vi "MoveXYAbs2.vi"(8 "error in (no error)":errorcluster, 9 "Y":dbl, 10 "X":dbl, 11 "connection ID":refnum<k5>) -> (0 "error out":errorcluster, 3 "connection ID 2":refnum<k5>)   [LabVIEW 2018]
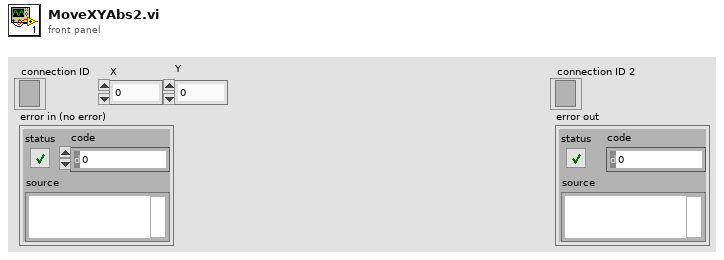
[diagram p1: front panel]
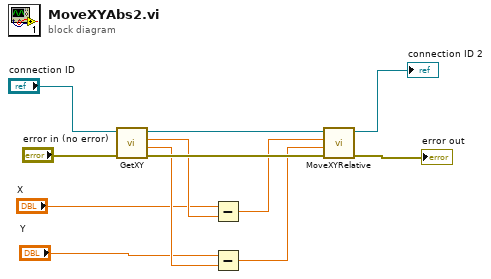
[diagram p0: block diagram]
diagram:
  n1 = call "GetXY.vi"("error in (no error)"="error in (no error)", "connection ID"="connection ID") -> ("error out"=w8:errorcluster, "Y"=w4:dbl, "X"=w5:dbl, "connection ID out"=w12:refnum<k5>)  [unwired: 6 in]
  n2 = Subtract(x="X", y=w5) -> (x-y=w7:dbl)
  n3 = Subtract(x="Y", y=w4) -> (x-y=w6:dbl)
  n4 = call "MoveXYRelative.vi"("error in (no error)"=w8, "Y"=w6, "X"=w7, "connection ID"=w12) -> ("error out"=→"error out":errorcluster, "connection ID 2"=→"connection ID 2":refnum<k5>)  [unwired: 6 in]
